vi "Check Action.vi"(6 "HRS Time":dbl, 8 "error in (no error)":errorcluster, 11 "Valve in":refnum<class "Valve.lvclass">) -> (0 "error out":errorcluster, 1 "Do Action":bool, 2 "Action":T1, 3 "Valve out":refnum<class "Valve.lvclass">)   [LabVIEW 2020, in "VolatusControl.lvlib" / "Valve.lvclass"]
uses:
  Valve.lvclass
  Valve.lvclass/Valve.ctl
  Volatus/MessageQ/MessageQ.lvclass
  Valve Action.ctl
  VolatusControl.lvlib
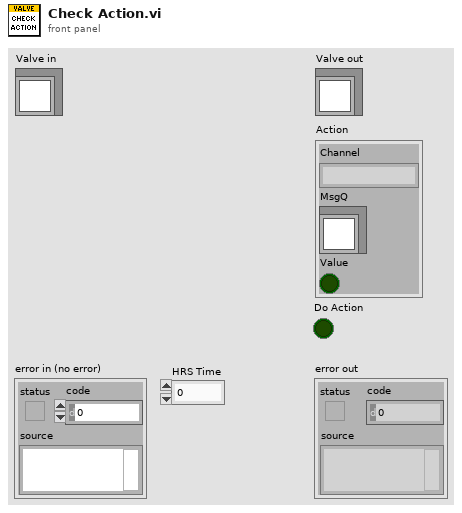
[diagram p1: front panel]
types:
  T1 = typedef "VolatusControl.lvlib/Valve Action.ctl" = cluster{"Channel":string, "MsgQ":refnum<class "MessageQ.lvclass">, "Value":bool}
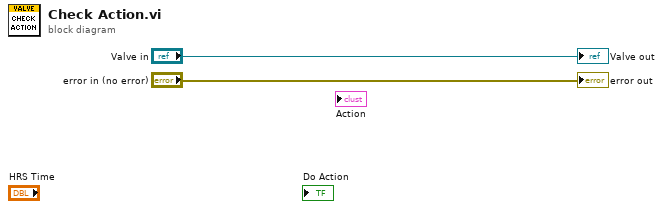
[diagram p0: block diagram]
diagram:
  "error out" <- "error in (no error)"
  "Valve out" <- "Valve in"
